vi "build request.vi"(8 "error in (no error)":errorcluster, 9 "JSON data":string="{\"fun_name\":\"myfunc\"}", 10 "binary data":u8[](array[numeric])=[1, 2, 3, 4], 11 "Command":T1=99 items=["async call"=97, "call function"=99, "ping"=112, "stop"=115, "unused"=254]) -> (0 "error out":errorcluster, 3 "REQ string":string)   [LabVIEW 2018, in "LV2Julia_core.lvlib"]
uses:
  LV2Julia_core.lvlib
  commands LV2Jl.ctl
  <vilib>/Utility/error.llb/Error Cluster From Error Code.vi
  <vilib>/ErrorRing/Error Ring.xnode
panel:
  out "REQ as byte arr":u8[](array[numeric]) format="%x"
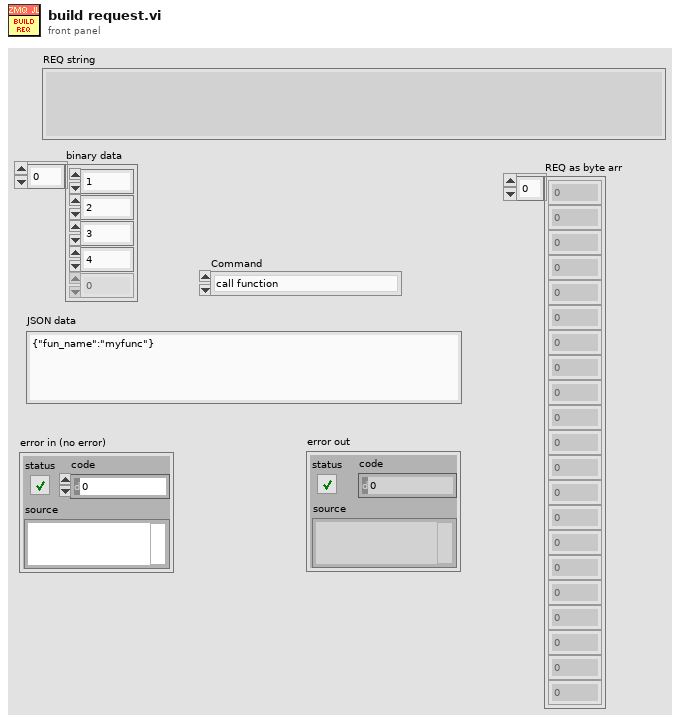
[diagram p1: front panel]
types:
  T1 = typedef "LV2Julia_core.lvlib/commands LV2Jl.ctl" = u8
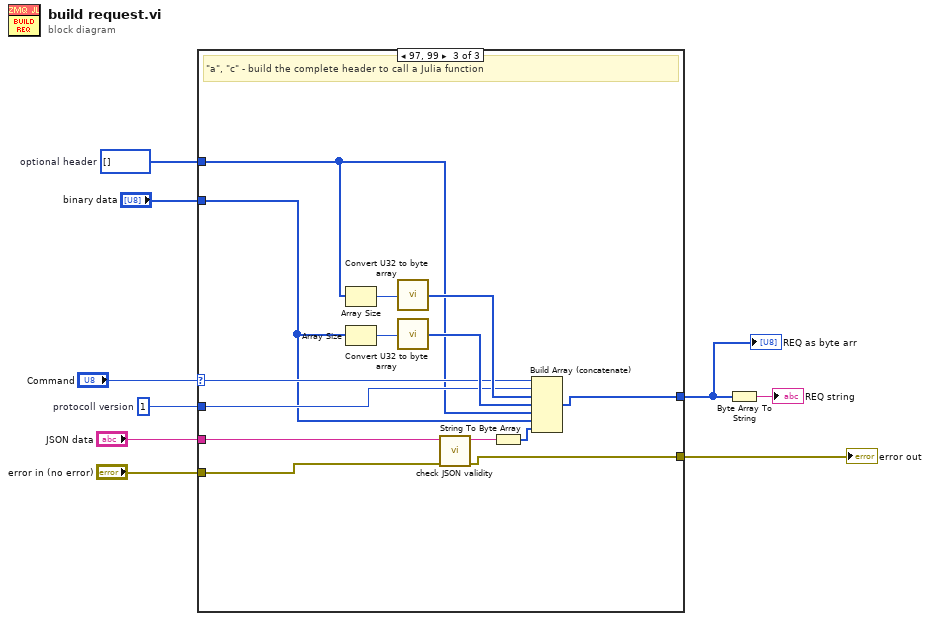
[diagram p0: block diagram]
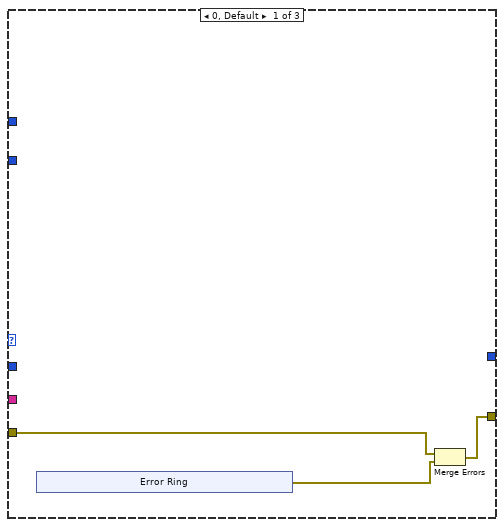
[diagram p2: hidden frame]
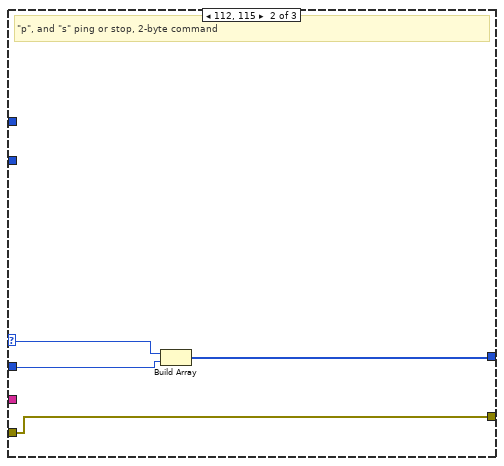
[diagram p3: hidden frame]
diagram:
  w6 = u8[] []  # optional header
  w1 = u8 1  # protocoll version
  n1 = case shown="97, 99" "Command" {
    selector: "Command" -> [_ w19 w27]
    tunnel: [w11 w21 w23] -> w9
    tunnel: [_ w18 w22] -> w8
    tunnel: w6 -> [_ _ w25]
    tunnel: "binary data" -> [_ _ w24]
    tunnel: "error in (no error)" -> [w10 w21 w29]
    tunnel: "JSON data" -> [_ _ w28]
    tunnel: w1 -> [_ w20 w26]
    frame 0, Default {
      n2 = xnode "Error Ring"() -> ("error out"=w12:errorcluster)
      n3 = Merge Errors(w10, w12) -> (w11:errorcluster)
    }
    frame 112, 115 {
      # "\"p\", and \"s\" ping or stop, 2-byte command"
      n4 = Build Array(w19, w20) -> (w18:T1[])
    }
    frame 97, 99 {
      # "\"a\", \"c\" - build the complete header to call a Julia function"
      n5 = Array Size(array=w25) -> (size(s)=w34:i32)
      n6 = Array Size(array=w24) -> (size(s)=w32:i32)
      n7 = call "Convert U32 to byte array.vi"("U32 in"=w34) -> ("Array of 4 bytes out"=w35:u8[])
      n8 = call "Convert U32 to byte array.vi"("U32 in"=w32) -> ("Array of 4 bytes out"=w33:u8[])
      n9 = call "check JSON validity.vi"("error in (no error)"=w29, "JSON string in"=w28) -> ("error out"=w23:errorcluster, "JSON string out"=w31:string)  [unwired: 8 in]
      n10 = String To Byte Array(string=w31) -> (unsigned byte array=w30:u8[])
      n11 = Build Array (concatenate)(w27, w26, w35, w33, w25, w24, w30) -> (w22:T1[])
    }
  }
  "error out" <- w9
  "REQ as byte arr" <- w8
  n12 = Byte Array To String(unsigned byte array=w8) -> (string=→"REQ string":string)
